vi "OL_command.vi"(8 "Sine (L)/Square (R)":bool, 9 "elapse time":dbl format="%0.2f", 10 "Amplitude":dbl=300.0, 11 "Frequency":dbl=0.5) -> (0 "Command Signal Graph":dbl[](graph)=[-300.0], 3 "Command Signal":dbl=-300.0)   [LabVIEW 2022 SP3]
uses:
  <vilib>/ptbypt/NI_PtbyPt.lvlib
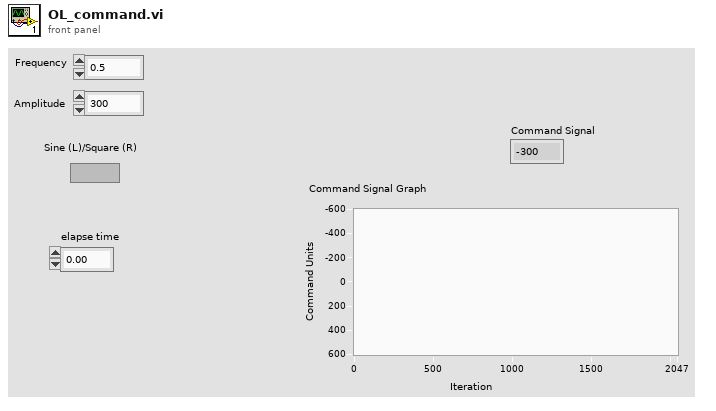
[diagram p1: front panel]
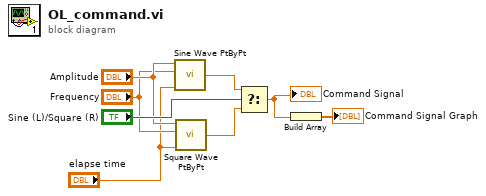
[diagram p0: block diagram]
diagram:
  n1 = call <vilib>:"Sine Wave PtByPt.vi"("time"="elapse time", "frequency"="Frequency", "amplitude"="Amplitude") -> ("sine wave"=w8:dbl)  [unwired: 1 in]
  n2 = call <vilib>:"Square Wave PtByPt.vi"("amplitude"="Amplitude", "frequency"="Frequency", "time"="elapse time") -> ("square wave"=w7:dbl)  [unwired: 2 in]
  n3 = Select(t=w8, s="Sine (L)/Square (R)", f=w7) -> (s? t:f=w1:dbl)
  "Command Signal" <- w1
  n4 = Build Array(w1) -> (→"Command Signal Graph":dbl[])
